vi "Colormap.vi"() -> (2 "Array":u32[](array[numeric]) format="%06x")   [LabVIEW 2012]
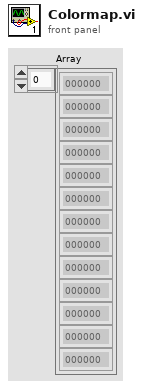
[diagram p1: front panel]
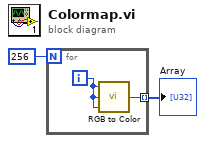
[diagram p0: block diagram]
diagram:
  n1 = for {
    N: 256 -> [_]
    tunnel: [w3] -> w1 mode=indexing
    i -> [w4]
    n2 = call <vilib>:"RGB to Color.vi"("B"=w4, "G"=w4, "R"=w4) -> ("Color"=w3:u32)
  }
  "Array" <- w1
